vi "Rupture.vi"(9 "(N0-N+1/N) dF/dt (pN/s)":dbl[](array[numeric]), 10 "Frupt (pN)":dbl[](array[numeric])) -> (1 "Fit result":string[][](array[string]), 2 "best nonlinear fit":dbl[](array[numeric]), 3 "Rupture analysis":cluster{dbl[], "Best Linear Fit":dbl[]}[](graph))   [LabVIEW 2018]
uses:
  <vilib>/gmath/NumericalOptimization/Nonlinear Curve Fit LM bound.vi
  <vilib>/gmath/NI_Gmath.lvlib
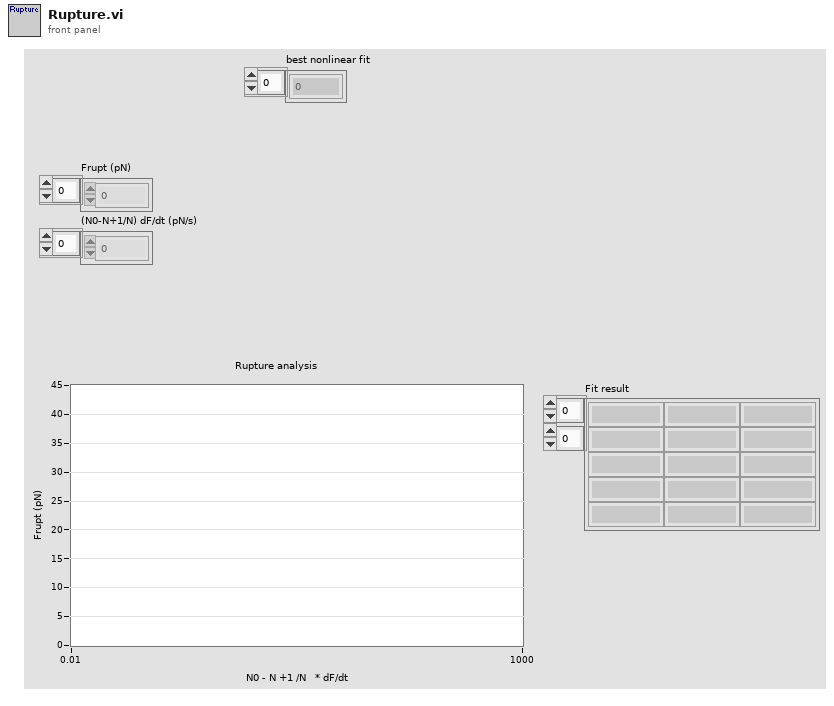
[diagram p1: front panel]
types:
  T1 = cluster{"parameter minimum":dbl[], "parameter maximum":dbl[]}
  T2 = typedef "NI_Matrix.lvlib/RealMatrix.ctl" = dbl[][]
  T3 = cluster{"(N0-N+1/N) dF/dt (pN/s)":dbl[], "Frupt (pN)":dbl[]}
  T4 = cluster{"(N0-N+1/N) dF/dt (pN/s)":dbl[], "best nonlinear fit":dbl[]}
  T5 = cluster{"(N0-N+1/N) dF/dt (pN/s)":dbl[], "best nonlinear fit":dbl[]}[]
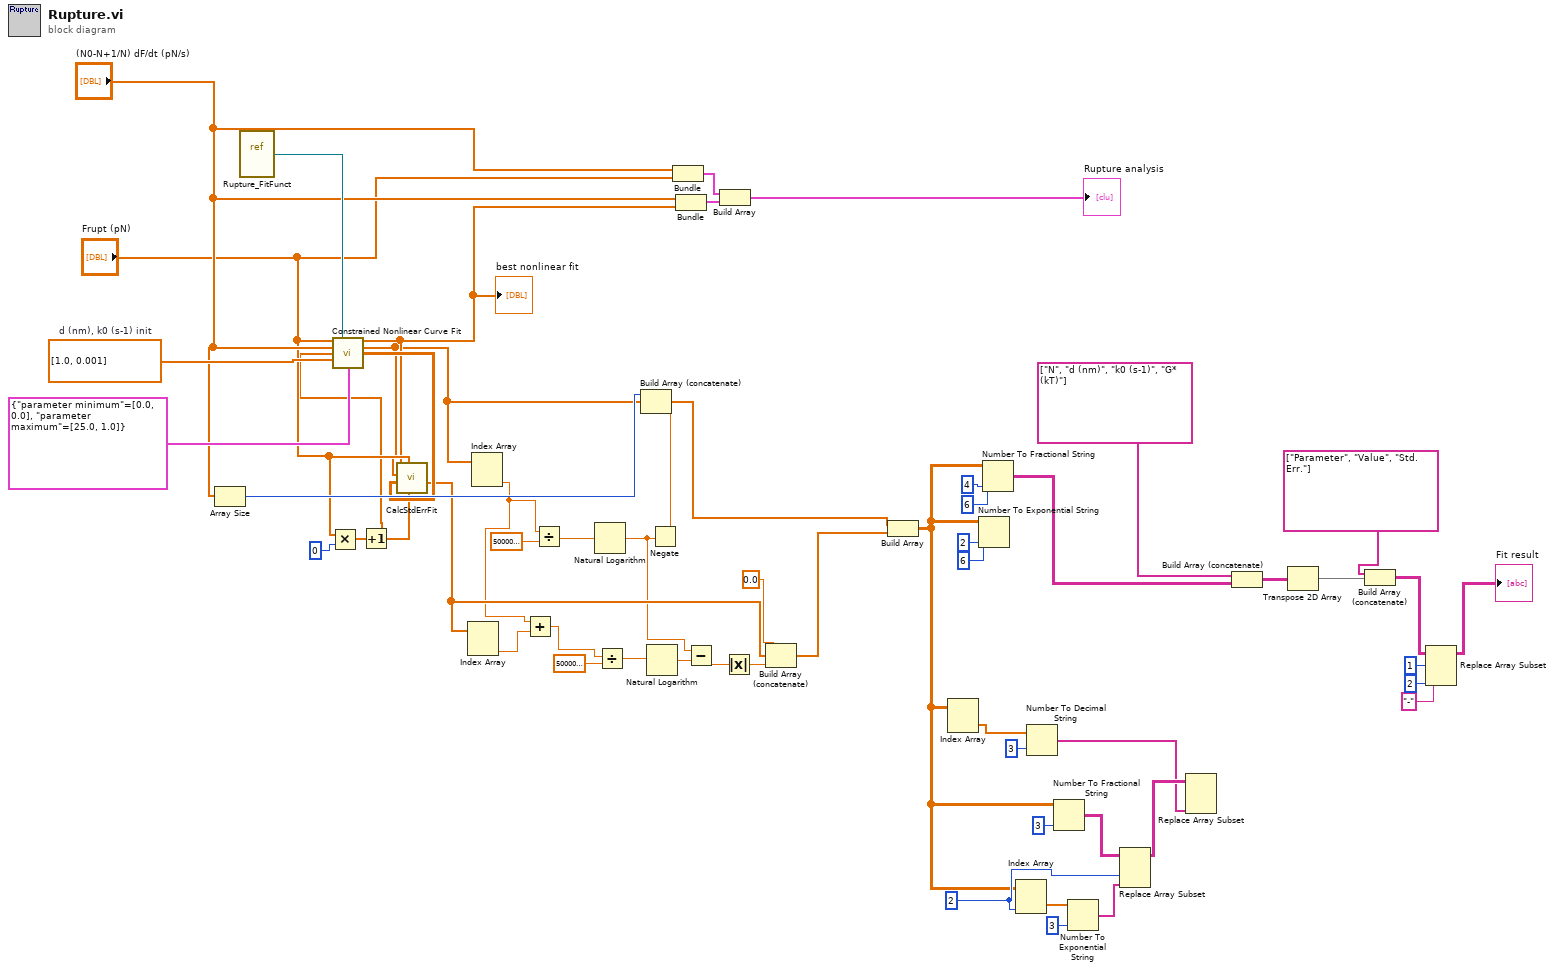
[diagram p0: block diagram]
diagram:
  w19 = 2 ("index (row)")
  w48 = dbl[] [1.0, 0.001]  # d (nm), k0 (s-1) init
  n1 = Array Size(array="(N0-N+1/N) dF/dt (pN/s)") -> (size(s)=w50:i32)
  n2 = vi-ref "Rupture_FitFunct.vi"() -> (w56:refnum<vi>)
  n3 = Multiply(x="Frupt (pN)", y=0) -> (x*y=w43:dbl[])
  n4 = Increment(x=w43) -> (x+1=w42:dbl[])
  n5 = call-poly <vilib>:"Constrained Nonlinear Curve Fit.vi"("Y"="Frupt (pN)", "f(x,a)"=w56, "X"="(N0-N+1/N) dF/dt (pN/s)", "Weight"=w42, "initial parameters"=w48, "parameter bounds"=T1 {"parameter minimum"=[0.0, 0.0], "parameter maximum"=[25.0, 1.0]}) -> ("best nonlinear fit"=w41:dbl[], "best fit parameters"=w40:dbl[], "covariance"=w47:T2)  [unwired: 4 in, 3 out]
  "best nonlinear fit" <- w41
  n6 = call "CalcStdErrFit.vi"("Weight"=w42, "Y"="Frupt (pN)", "covariance"=w47, "Best Fit Params"=w40, "best nonlinear fit"=w41) -> ("std error"=w37:dbl[])  [unwired: 4 in, 2 out]
  n7 = Index Array(array=w37) -> (element #2=w14:dbl)  [unwired: 2 in, 1 out]
  n8 = Index Array(array=w40) -> (element #2=w15:dbl)  [unwired: 2 in, 1 out]
  n9 = Add(x=w15, y=w14) -> (x+y=w13:dbl)
  n10 = Divide(x=w15, y=5000000000.0) -> (x/y=w54:dbl)
  n11 = Natural Logarithm(1:w54) -> (0:w8:dbl)
  n12 = Divide(x=w13, y=5000000000.0) -> (x/y=w38:dbl)
  n13 = Natural Logarithm(1:w38) -> (0:w12:dbl)
  n14 = Negate(x=w8) -> (-x=w11:dbl)
  n15 = Build Array (concatenate)(w50, w40, w11) -> (w35:dbl[])
  n16 = Bundle("(N0-N+1/N) dF/dt (pN/s)"="(N0-N+1/N) dF/dt (pN/s)", "Frupt (pN)"="Frupt (pN)") -> (w51:T3)  [unwired: 1 in]
  n17 = Bundle("(N0-N+1/N) dF/dt (pN/s)"="(N0-N+1/N) dF/dt (pN/s)", "best nonlinear fit"=w41) -> (w53:T4)  [unwired: 1 in]
  n18 = Subtract(x=w8, y=w12) -> (x-y=w9:dbl)
  n19 = Build Array(w51, w53) -> (→"Rupture analysis":T5)
  n20 = Absolute Value(x=w9) -> (abs(x)=w10:dbl)
  n21 = Build Array (concatenate)(0.0 ("element"), w37, w10) -> (w34:dbl[])
  n22 = Build Array(w35, w34) -> (w4:dbl[][])
  n23 = Index Array(array=w4) -> (element=w18:dbl[])  [unwired: 2 in]
  n24 = Number To Exponential String(number=w4, precision (6)=i16 2, 3:i16 6 ("width (-)")) -> ()  [unwired: 1 in, 1 out]
  n25 = Number To Fractional String(number=w4, width (-)=i16 6, precision (6)=i16 4 ("width (-)")) -> (F-format string=w2:string[][])  [unwired: 1 in]
  n26 = Index Array(array=w4, index (col)=w19) -> (element=w23:dbl[])  [unwired: 1 in]
  n27 = Number To Decimal String(number=w18, width (-)=i16 3) -> (decimal integer string=w16:string[])
  n28 = Number To Fractional String(number=w4, precision (6)=i16 3) -> (F-format string=w22:string[][])  [unwired: 2 in]
  n29 = Number To Exponential String(number=w23, precision (6)=i16 3) -> (E-format string=w21:string[])  [unwired: 2 in]
  n30 = Replace Array Subset(array=w22, new element=w21, index (col)=w19) -> (w17:string[][])  [unwired: 1 in]
  n31 = Replace Array Subset(array=w17, new element=w16) -> ()  [unwired: 2 in, 1 out]
  n32 = Build Array (concatenate)(string[] ["N", "d (nm)", "k0 (s-1)", "G* (kT)"] ("element"), w2) -> (w32:string[][])
  n33 = Transpose 2D Array(2D array=w32) -> (transposed array=w31:string[][])
  n34 = Build Array (concatenate)(string[] ["Parameter", "Value", "Std. Err."] ("element"), w31) -> (w28:string[][])
  n35 = Replace Array Subset(array=w28, new element="-" ("new element/subarray"), index (row)=1, index (col)=2 ("disabled index (col)")) -> (→"Fit result":string[][])
